vi "Store Arbitrary Waveform.vi"(8 "error in (no error)":errorcluster, 9 "File Path (INT:\\test.arb)":string="INT:\\test.arb", 10 "Channel (1: 1)":i32(ring)=1 items=["1"=1, "2"=2], 11 "VISA resource name":refnum<visa-resource-name>) -> (0 "error out":errorcluster, 3 "VISA resource name out":refnum<visa-resource-name>)   [LabVIEW 2026, in "Agilent 3352X Series.lvlib"]
doc: "Stores current loaded arb segment(.arb/.barb) or arb sequence (.seq) data in the channel specified volatile memory to INTERNAL or USB memory"
uses:
  Agilent 3352X Series.lvlib
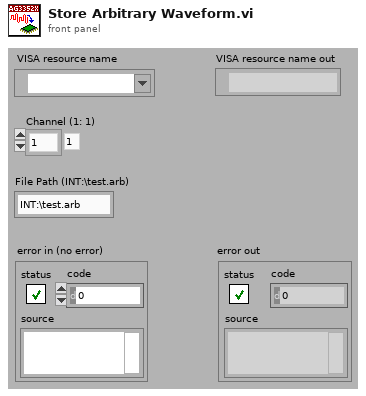
[diagram p1: front panel]
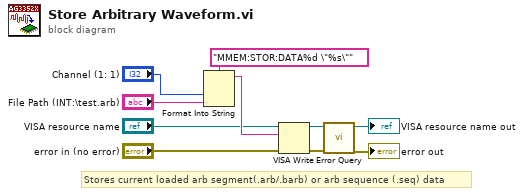
[diagram p0: block diagram]
diagram:
  # "Stores current loaded arb segment(.arb/.barb) or arb sequence (.seq) data"
  n1 = Format Into String(format string="MMEM:STOR:DATA%d \"%s\"", "Channel (1: 1)", "File Path (INT:\\test.arb)") -> (resulting string=w7:string)  [unwired: 2 in, 1 out]
  n2 = VISA Write(VISA resource name="VISA resource name", write buffer=w7, error in (no error)="error in (no error)") -> (VISA resource name out=w4:refnum<visa-resource-name>, error out=w3:errorcluster)  [unwired: 1 out]
  n3 = call "Error Query.vi"("error in (no error)"=w3, "VISA resource name"=w4) -> ("error out"=→"error out":errorcluster, "VISA resource name out"=→"VISA resource name out":refnum<visa-resource-name>)  [unwired: 8 out]
